vi "Cal Plot Scale.vi"(8 "error in (no error)":errorcluster, 11 "Domain in":refnum<class "NI_Domain.lvclass">) -> (0 "error out":errorcluster, 1 "Y Scale":T1, 2 "X Scale":T1, 3 "Domain out":refnum<class "NI_Domain.lvclass">, 4 "# of t-points":i32)   [LabVIEW 2017, in "NI_PDE.lvlib" / "NI_Domain.lvclass"]
uses:
  <vilib>/gmath/pde.llb/DomainClass/NI_Domain.lvclass
  <vilib>/Utility/miscctls.llb/LVOffsetAndMultiplierTypeDef.ctl
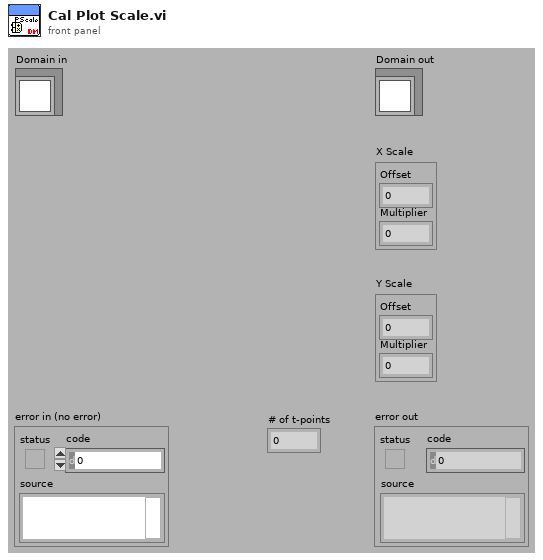
[diagram p1: front panel]
types:
  T1 = typedef "LVOffsetAndMultiplierTypeDef.ctl" = cluster{"Offset":dbl, "Multiplier":dbl}
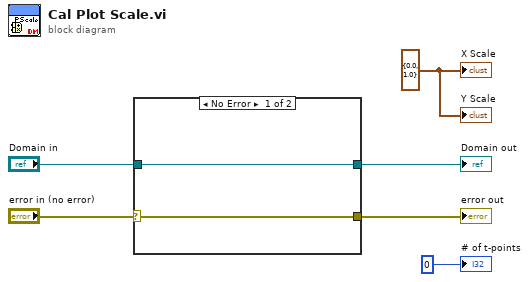
[diagram p0: block diagram]
diagram:
  w1 = T1 {"Offset"=0.0, "Multiplier"=1.0} ("X Scale")
  n1 = case shown="No Error" "error in (no error)" {
    selector: "error in (no error)" -> [w7 w10]
    tunnel: "Domain in" -> [w8 w9]
    tunnel: [w8 w9] -> w6
    tunnel: [w7 w10] -> w5
    frame No Error {
    }
    frame Error {
    }
  }
  "Domain out" <- w6
  "error out" <- w5
  "X Scale" <- w1
  "Y Scale" <- w1
  "# of t-points" <- 0 ("# of t-points")
